vi "模拟量输入自动测试一组_fast_OK.vi"(8 "AD选择？":bool, 9 "DSP选择？":bool, 11 "第几个":i32) -> ()   [LabVIEW 2010]
uses:
  全局量/试验配置信息.vi
panel:
  in  "AD测试值":dbl[](array[numeric])
  in  "DSP测试值":dbl[](array[numeric])
  # "从0开始"
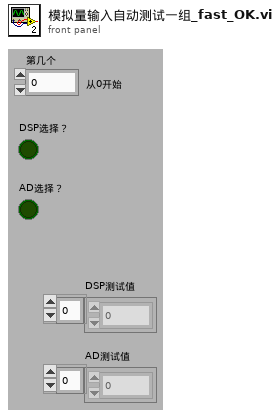
[diagram p1: front panel]
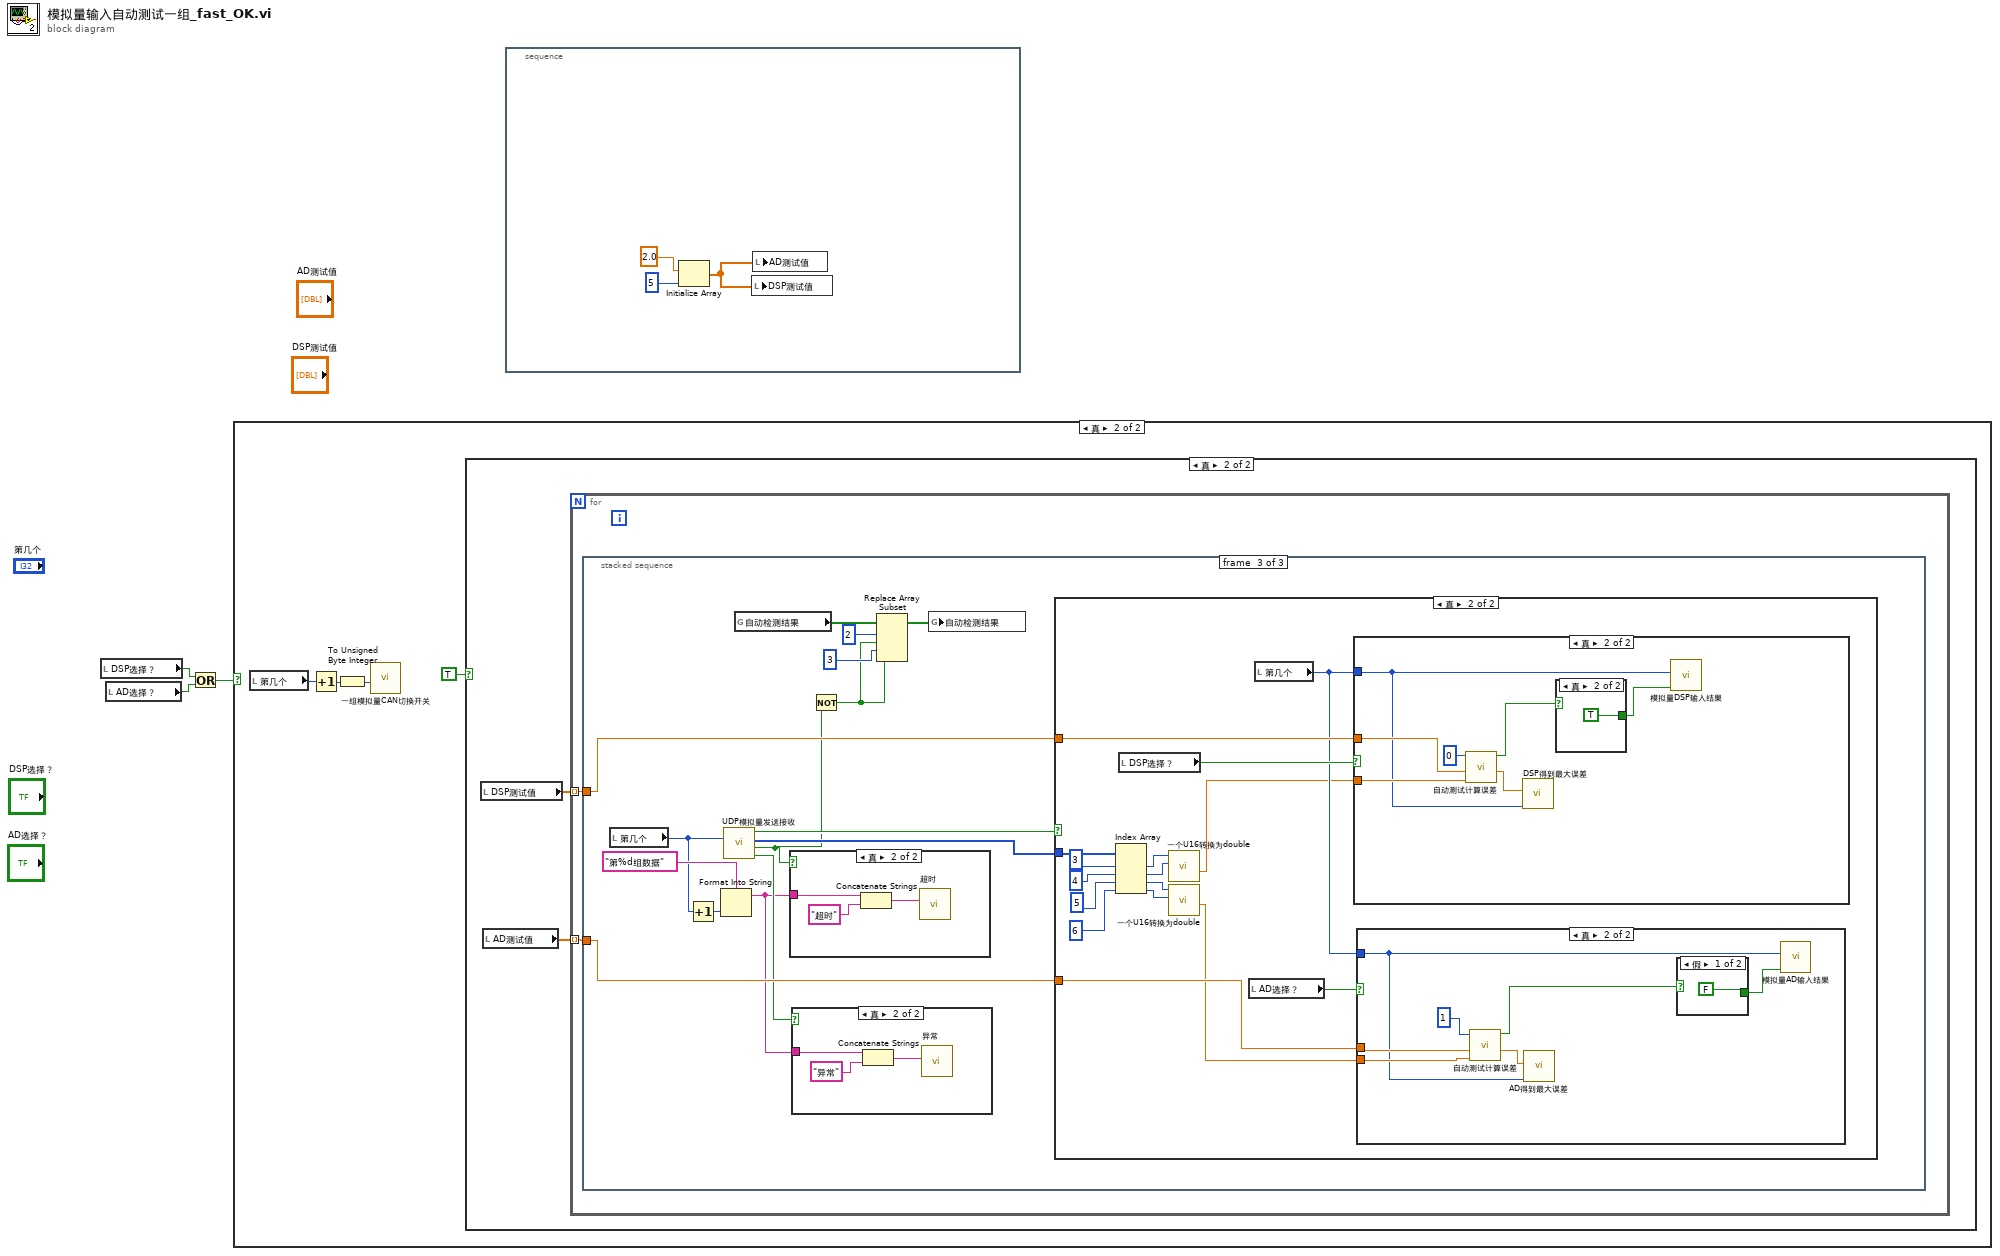
[diagram p0: block diagram]
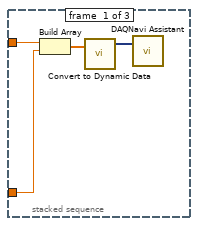
[diagram p4: hidden frame]
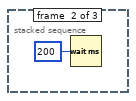
[diagram p5: hidden frame]
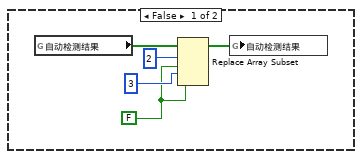
[diagram p8: hidden frame]
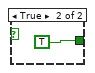
[diagram p10: hidden frame]
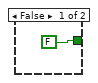
[diagram p12: hidden frame]
diagram:
  n1 = local read "DSP选择？"() -> (w2:bool)
  n2 = local read "AD选择？"() -> (w3:bool)
  n3 = Or(x=w2, y=w3) -> (x .or. y?=w1:bool)
  n4 = case shown="真" w1 {
    frame False {
    }
    frame True {
      n5 = local read "第几个"() -> (w7:i32)
      n6 = Increment(x=w7) -> (x+1=w5:i32)
      n7 = To Unsigned Byte Integer(number=w5) -> (unsigned 8bit integer=w6:u8)
      n8 = call "一组模拟量CAN切换开关.vi"("第几组数据"=w6) -> ()  [unwired: 10 in, 1 out]
      n9 = case shown="真" TRUE {
        frame False {
        }
        frame True {
          n10 = local read "DSP测试值"() -> (w9:dbl[])
          n11 = local read "AD测试值"() -> (w8:dbl[])
          n12 = for {
            tunnel: w9 -> [w11] mode=indexing
            tunnel: w8 -> [w10] mode=indexing
            n13 = stacked-sequence {
              tunnel: w11 -> [w13 _ w31]
              tunnel: w10 -> [w12 _ w30]
              frame #0 {
                n14 = Build Array(w13, w12) -> (w15:dbl[])
                n15 = call "Convert to Dynamic Data"("Array"=w15) -> ("Dynamic Data Type"=w14:dynamicdata)  [unwired: 3 out]
                n16 = call "DAQNavi Assistant"("data in(DDT)"=w14) -> ()  [unwired: 2 in, 17 out]
              }
              frame #1 {
                n17 = Wait (ms)(milliseconds to wait=u32 200 ("等待时间（毫秒）")) -> ()  [unwired: 1 out]
              }
              frame #2 {
                n18 = local read "第几个"() -> (w23:i32)
                n19 = Increment(x=w23) -> (x+1=w24:i32)
                n20 = Format Into String(format string="第%d组数据" ("格式字符串"), w24) -> (resulting string=w25:string)  [unwired: 2 in, 1 out]
                n21 = call "UDP模拟量发送接收.vi"("第几组"=w23) -> ("异常_找到?"=w26:bool, "接收超时?"=w19:bool, "接收的一帧数据"=w29:u16[], "正常_找到?"=w28:bool)  [unwired: 7 in]
                n22 = global read "试验配置信息.vi" "自动检测结果"() -> (w20:bool[])
                n23 = case shown="真" w19 {
                  tunnel: w25 -> [_ w37]
                  frame False {
                  }
                  frame True {
                    n24 = Concatenate Strings(w37, "超时" ("格式字符串")) -> (w35:string)
                    n25 = call "超时"("Message"=w35) -> ()  [unwired: 9 in, 2 out]
                  }
                }
                n26 = case shown="真" w26 {
                  tunnel: w25 -> [_ w34]
                  frame False {
                  }
                  frame True {
                    n27 = Concatenate Strings(w34, "异常" ("格式字符串")) -> (w32:string)
                    n28 = call "异常"("Message"=w32) -> ()  [unwired: 9 in, 2 out]
                  }
                }
                n29 = Not(x=w19) -> (.not. x?=w17:bool)
                n30 = Replace Array Subset(array=w20, new element #1=w17, index #1=2 ("索引"), new element #2=w17, index #2=3 ("索引")) -> (w21:bool[])
                n31 = global write "试验配置信息.vi" "自动检测结果"(w21) -> ()
                n32 = case shown="真" w28 {
                  tunnel: w29 -> [_ w50]
                  tunnel: w31 -> [_ w48]
                  tunnel: w30 -> [_ w47]
                  frame False {
                    w38 = FALSE
                    n33 = global read "试验配置信息.vi" "自动检测结果"() -> (w41:bool[])
                    n34 = Replace Array Subset(array=w41, new element #1=w38, index #1=2 ("索引"), new element #2=w38, index #2=3 ("索引")) -> (w40:bool[])
                    n35 = global write "试验配置信息.vi" "自动检测结果"(w40) -> ()
                  }
                  frame True {
                    n36 = Index Array(array=w50, index #1=3 ("索引"), index #2=4 ("索引"), index #3=5 ("索引"), index #4=6 ("索引")) -> (element #1=w55:u16, element #2=w56:u16, element #3=w57:u16, element #4=w58:u16)
                    n37 = local read "DSP选择？"() -> (w49:bool)
                    n38 = call "一个U16转换为double.vi"("低16位_1"=w56, "高16位_1"=w55) -> ("反馈值"=w43:dbl)  [unwired: 9 in]
                    n39 = call "一个U16转换为double.vi"("低16位_1"=w58, "高16位_1"=w57) -> ("反馈值"=w46:dbl)  [unwired: 9 in]
                    n40 = local read "AD选择？"() -> (w45:bool)
                    n41 = local read "第几个"() -> (w44:i32)
                    n42 = case shown="真" w49 {
                      tunnel: w48 -> [_ w73]
                      tunnel: w43 -> [_ w72]
                      tunnel: w44 -> [_ w68]
                      frame False {
                      }
                      frame True {
                        n43 = call "自动测试计算误差.vi"("反馈值"=w72, "输入值"=w73, "DSP_OR_AD"=0) -> ("误差"=w69:dbl, "合格？"=w71:bool)  [unwired: 7 in]
                        n44 = call "DSP得到最大误差.vi"("第几组"=w68, "新误差值"=w69) -> ()  [unwired: 10 in]
                        n45 = case shown="真" w71 {
                          tunnel: [FALSE TRUE] -> w70
                          frame False {
                          }
                          frame True {
                          }
                        }
                        n46 = call "模拟量DSP输入结果.vi"("合格?"=w70, "第几个"=w68) -> ()  [unwired: 10 in]
                      }
                    }
                    n47 = case shown="真" w45 {
                      tunnel: w47 -> [_ w63]
                      tunnel: w46 -> [_ w62]
                      tunnel: w44 -> [_ w59]
                      frame False {
                      }
                      frame True {
                        n48 = call "自动测试计算误差.vi"("反馈值"=w62, "输入值"=w63, "DSP_OR_AD"=1) -> ("误差"=w60:dbl, "合格？"=w64:bool)  [unwired: 7 in]
                        n49 = call "AD得到最大误差.vi"("第几组"=w59, "新误差值"=w60) -> ()  [unwired: 10 in]
                        n50 = case shown="假" w64 {
                          tunnel: [FALSE TRUE] -> w61
                          frame False {
                          }
                          frame True {
                          }
                        }
                        n51 = call "模拟量AD输入结果.vi"("合格?"=w61, "第几个"=w59) -> ()  [unwired: 10 in]
                      }
                    }
                  }
                }
              }
            }
          }
        }
      }
    }
  }
  n52 = stacked-sequence {
    frame #0 {
      n53 = Initialize Array(2.0, 5 ("维数大小")) -> (w77:dbl[])
      n54 = local write "DSP测试值"(w77) -> ()
      n55 = local write "AD测试值"(w77) -> ()
    }
  }
